vi "API String - Float Precision.vi"(8 "Error in":errorcluster caption="Error in (no error)") -> (0 "Error out":errorcluster, 3 "Precision":u8)   [LabVIEW 2017, in "API String Arguments Support.lvlib"]
uses:
  API String Arguments Support.lvlib
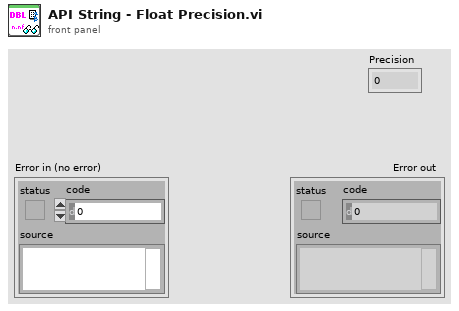
[diagram p1: front panel]
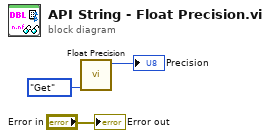
[diagram p0: block diagram]
diagram:
  n1 = call "Float Precision.vi"("Enum"=enum16{"Set", "Get"}."Get") -> ("Precision out"=→"Precision":u8)  [unwired: 9 in, 1 out]
  "Error out" <- "Error in"
